vi "InitializePlayerDataFolder.vi"(8 "error in (no error)":errorcluster, 9 "BaseDataFolder":path, 10 "Player in":refnum<class "Player.lvclass">) -> (0 "error out":errorcluster, 1 "PlayerDataPath":path, 2 "Player out":refnum<class "Player.lvclass">)   [LabVIEW 2015, in "TronviewGame.lvlib" / "Game.lvclass"]
uses:
  Game.lvclass
  Player/Player.lvclass
  Player/Player.lvclass/Player.ctl
  Player/GetPlayerName.vi
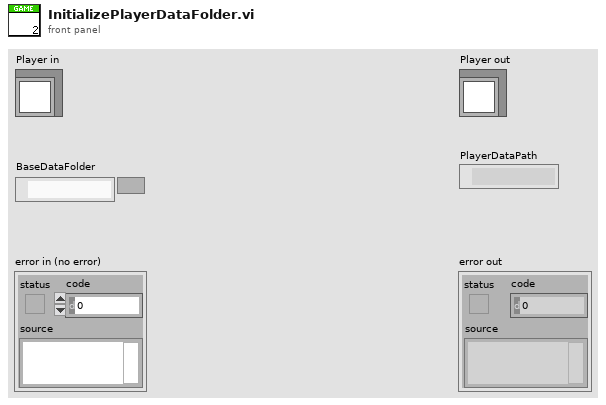
[diagram p1: front panel]
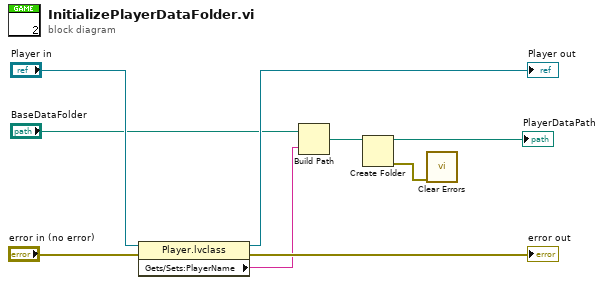
[diagram p0: block diagram]
diagram:
  n1 = property class="Player.lvclass"(reference="Player in", error in="error in (no error)") -> (reference out=→"Player out":refnum<class "Player.lvclass">, error out=→"error out":errorcluster, "Gets/Sets:PlayerName"=w4:string)
  n2 = Build Path(base path="BaseDataFolder", name or relative path=w4) -> (appended path=w3:path)
  n3 = Create Folder(path (use dialog)=w3) -> (created path=→"PlayerDataPath":path, error out=w2:errorcluster)  [unwired: 2 in, 1 out]
  n4 = call <vilib>:"Clear Errors.vi"("error in (no error)"=w2) -> ()  [unwired: 5 in, 2 out]
